vi "PrepareView.vi"(8 "error in":errorcluster, 10 "ICellVirtual":refnum<k24>, 11 "Cell View Back Color Alternate in":refnum<class "Cell View Back Color Alternate.lvclass">) -> (0 "error out":errorcluster, 3 "Cell View Back Color Alternate out":refnum<class "Cell View Back Color Alternate.lvclass">)   [LabVIEW 2024, in "PDO Grid.lvlib" / "Cell View Back Color Alternate.lvclass"]
uses:
  Cell View Back Color Alternate.lvclass
  Cell View Back Color Alternate.lvclass/Cell View Back Color Alternate.ctl
  Sourcegrid-LabVIEW/source/Color/Color.lvclass/Color.ctl
  D:/git/Sourcegrid-LabVIEW/dll/SourceGrid.dll
  Sourcegrid-LabVIEW/dll/SourceGrid.dll
  Sourcegrid-LabVIEW/source/Color/Color.lvclass
  Sourcegrid-LabVIEW/source/Views/ViewBase/Cell View.lvclass
  D:/git/Sourcegrid-LabVIEW/source/Views/ViewBase/Cell View.lvclass
  D:/git/Sourcegrid-LabVIEW/source/ICloseable/ICloseable.lvclass
  D:/git/EDS-File-Viewer/source/Cell View Back Color Alternate/Cell View Back Color Alternate.lvclass
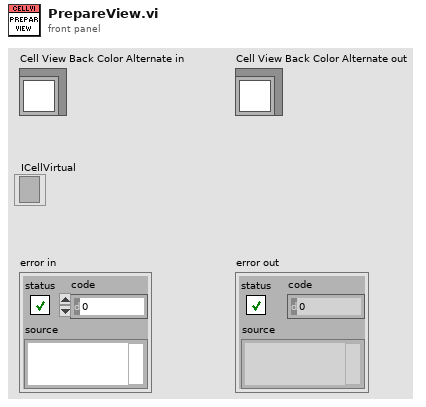
[diagram p1: front panel]
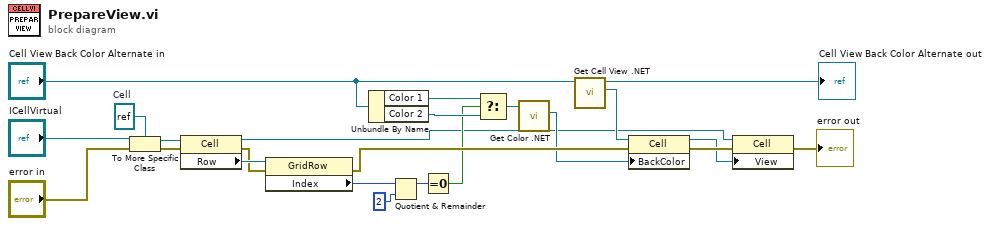
[diagram p0: block diagram]
diagram:
  w19 = refnum<k24> refnum  # Cell
  n1 = To More Specific Class(target class=w19, reference="ICellVirtual", error in="error in") -> (specific class reference=w20:refnum<k24>, error out=w22:errorcluster)
  n2 = property class="Cell"(reference=w20, error in=w22) -> (reference out=w1:refnum<k24>, error out=w16:errorcluster, "Row"=w18:refnum<k24>)
  n3 = property class="GridRow"(reference=w18, error in=w16) -> (error out=w13:errorcluster, "Index"=w17:i32)  [unwired: 1 out]
  n4 = Unbundle By Name("Cell View Back Color Alternate in") -> ("Color 1"=w11:refnum<class "Color.lvclass">, "Color 2"=w10:refnum<class "Color.lvclass">)
  n5 = Quotient & Remainder(x=w17, y=2) -> (x-y*floor(x/y)=w14:i32)  [unwired: 1 out]
  n6 = Equal To 0?(x=w14) -> (x = 0?=w8:bool)
  n7 = Select(t=w11, s=w8, f=w10) -> (s? t:f=w9:refnum<class "Color.lvclass">)
  n8 = call "Get Color .NET.vi"("Color in"=w9) -> ("Color .NET"=w7:refnum<k24>)  [unwired: 9 in, 1 out]
  n9 = call "Get Cell View .NET.vi"("Cell View in"="Cell View Back Color Alternate in") -> ("Cell View .NET"=w5:refnum<k24>, "Cell View out"=→"Cell View Back Color Alternate out":refnum<class "Cell View Back Color Alternate.lvclass">)  [unwired: 9 in]
  n10 = property class="Cell"(reference=w5, error in=w13, "BackColor"=w7) -> (reference out=w3:refnum<k24>, error out=w4:errorcluster)
  n11 = property class="Cell"(reference=w1, error in=w4, "View"=w3) -> (error out=→"error out":errorcluster)  [unwired: 1 out]
